vi "get_chemicals.vi"() -> ()   [LabVIEW 2018]
panel:
  in  "Diluent":string(combo)
  in  "Oxidizer":string(combo)
  in  "Fuel":string(combo)
  in  "stop":bool
  in  "Mechanism":string(combo)
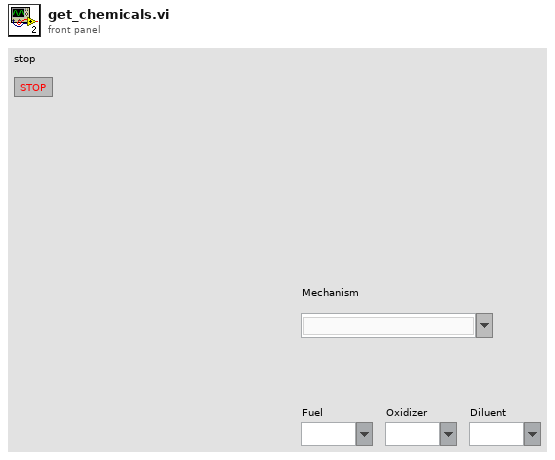
[diagram p1: front panel]
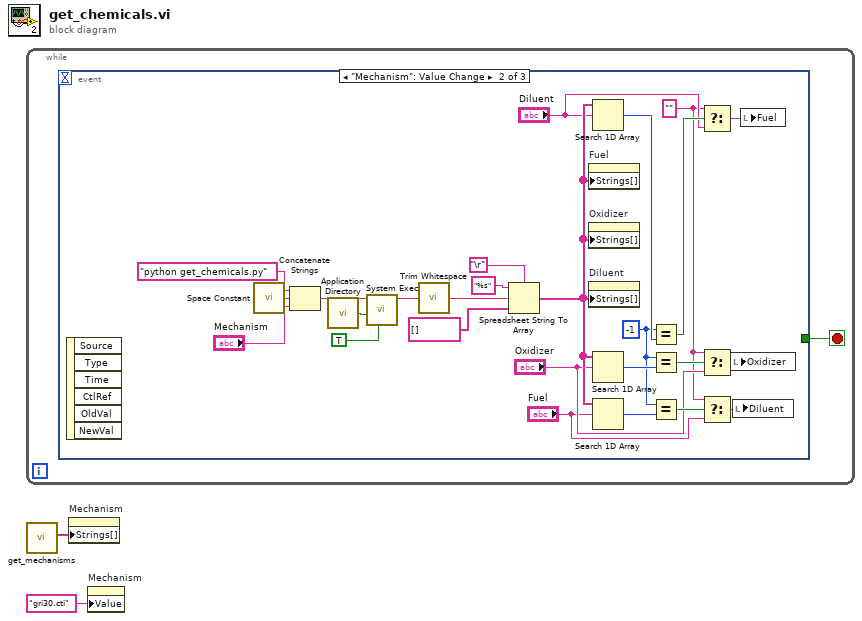
[diagram p0: block diagram]
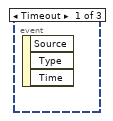
[diagram p2: hidden frame]
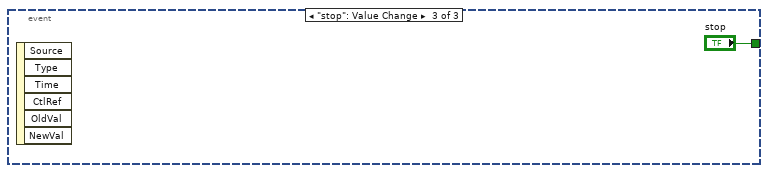
[diagram p3: hidden frame]
diagram:
  n1 = while {
    stop <- w3 stop-if-true
    n2 = event shown="[1] \"Mechanism\": Value Change" {
      selector: _ -> [_ _ _]
      dyn-events: _ -> [_ _ _]
      timeout: _ -> [_ _ _]
      tunnel: [_ _ "stop"] -> w3
      event Timeout {
        n3 = event-data() -> ()  [unwired: 1 in, 3 out]
      }
      event "Mechanism": Value Change {
        w7 = "" ("t")
        w14 = -1 ("x")
        n4 = event-data() -> ()  [unwired: 1 in, 6 out]
        n5 = call <vilib>:"Space Constant.vi"() -> ("String"=w28:string)
        n6 = Concatenate Strings("python get_chemicals.py" ("command line"), w28, "Mechanism") -> (w25:string)
        n7 = call <vilib>:"Application Directory.vi"() -> ("Application Directory"=w29:path)
        n8 = call <vilib>:"System Exec.vi"("run minimized? (F)"=TRUE, "working directory"=w29, "command line"=w25) -> ("standard output"=w24:string)  [unwired: 5 in, 3 out]
        n9 = call <vilib>:"Trim Whitespace.vi"("string"=w24) -> ("trimmed string"=w23:string)  [unwired: 1 in]
        n10 = Spreadsheet String To Array(delimiter (Tab)="\r", format string="%s", spreadsheet string=w23, array type (2D Dbl)=string[] []) -> (array=w18:string[])
        n11 = property on="Fuel" class="CmbBox"("Strings[]"=w18) -> ()  [unwired: 2 in, 2 out]
        n12 = property on="Oxidizer" class="CmbBox"("Strings[]"=w18) -> ()  [unwired: 2 in, 2 out]
        n13 = property on="Diluent" class="CmbBox"("Strings[]"=w18) -> ()  [unwired: 2 in, 2 out]
        n14 = Search 1D Array(1D array=w18, element="Diluent") -> (index of element=w15:i32)  [unwired: 1 in]
        n15 = Search 1D Array(1D array=w18, element="Oxidizer") -> (index of element=w16:i32)  [unwired: 1 in]
        n16 = Search 1D Array(1D array=w18, element="Fuel") -> (index of element=w17:i32)  [unwired: 1 in]
        n17 = Equal?(x=w14, y=w15) -> (x = y?=w11:bool)
        n18 = Equal?(x=w14, y=w16) -> (x = y?=w12:bool)
        n19 = Equal?(x=w14, y=w17) -> (x = y?=w13:bool)
        n20 = Select(t=w7, s=w11, f="Diluent") -> (s? t:f=w5:string)
        n21 = Select(t=w7, s=w12, f="Oxidizer") -> (s? t:f=w4:string)
        n22 = Select(t=w7, s=w13, f="Fuel") -> (s? t:f=w6:string)
        n23 = local write "Oxidizer"(w4) -> ()
        n24 = local write "Diluent"(w6) -> ()
        n25 = local write "Fuel"(w5) -> ()
      }
      event "stop": Value Change {
        n26 = event-data() -> ()  [unwired: 1 in, 6 out]
      }
    }
  }
  n27 = call "get_mechanisms.vi"() -> ("Mechanisms"=w1:string[])  [unwired: 11 in]
  n28 = property on="Mechanism" class="CmbBox"("Strings[]"=w1) -> ()  [unwired: 2 in, 2 out]
  n29 = property on="Mechanism" class="CmbBox"("Value"="gri30.cti") -> ()  [unwired: 2 in, 2 out]
